vi "opencvSelectSubset.vi"(0 "x0":dbl, 1 "dx":dbl, 2 "y0":dbl, 3 "dy":dbl, 4 "YX":u16[][](array[numeric])) -> (5 "Array":u16[][](array[numeric]))   [LabVIEW 2017]
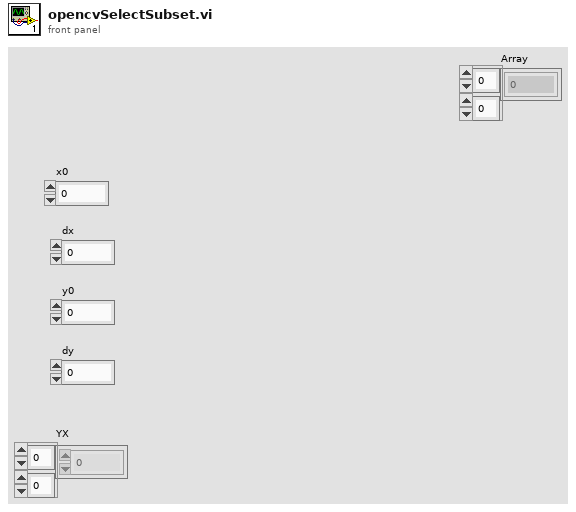
[diagram p1: front panel]
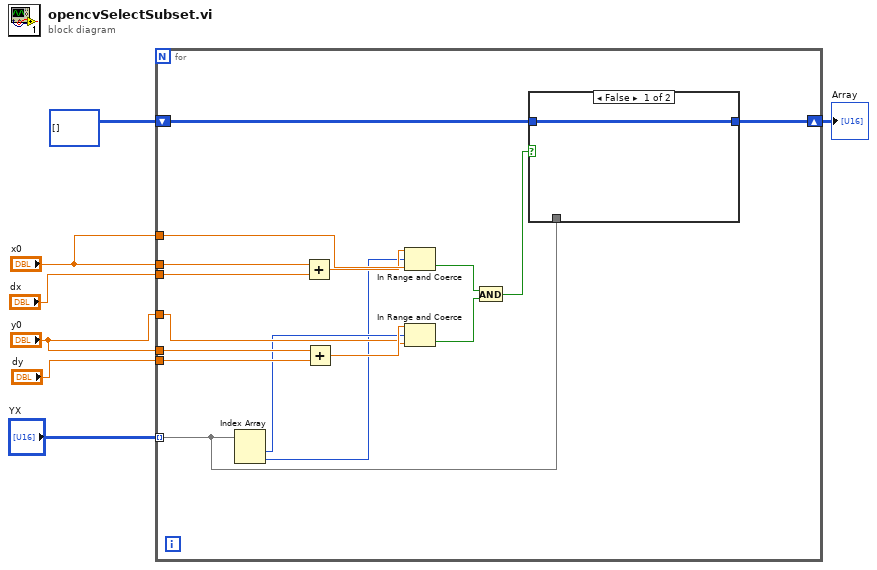
[diagram p0: block diagram]
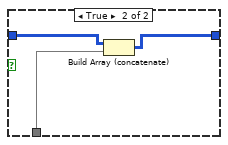
[diagram p2: hidden frame]
diagram:
  n1 = for {
    tunnel: "YX" -> [w10] mode=indexing
    tunnel: "x0" -> [w23]
    tunnel: "dx" -> [w22]
    tunnel: "x0" -> [w16]
    tunnel: "y0" -> [w21]
    tunnel: "dy" -> [w20]
    tunnel: "y0" -> [w18]
    shift-right: [w9] -> w1
    shift-left: u16[][] [] -> [w11]
    n2 = Index Array(array=w10) -> (element #1=w17:u16, element #2=w14:u16)  [unwired: 2 in]
    n3 = Add(x=w23, y=w22) -> (x+y=w15:dbl)
    n4 = Add(x=w21, y=w20) -> (x+y=w19:dbl)
    n5 = In Range and Coerce(upper limit=w15, x=w14, lower limit=w16) -> (In Range?=w13:bool)  [unwired: 1 out]
    n6 = In Range and Coerce(upper limit=w19, x=w17, lower limit=w18) -> (In Range?=w12:bool)  [unwired: 1 out]
    n7 = And(x=w13, y=w12) -> (x .and. y?=w8:bool)
    n8 = case shown="False" w8 {
      tunnel: w11 -> [w24 w27]
      tunnel: w10 -> [_ w26]
      tunnel: [w24 w25] -> w9
      frame False {
      }
      frame True {
        n9 = Build Array (concatenate)(w27, w26) -> (w25:u16[][])
      }
    }
  }
  "Array" <- w1
